vi "TrigerDelayer_测试Main.vi"() -> ()   [LabVIEW 2016]
uses:
  TrigerDelayer_ctl_TriggerSource.ctl
  Trigger Delayer.lvlib
panel:
  in  "Cluster":T2
  out "error out":errorcluster
  out "VISA resource name out":refnum<visa-resource-name>
  in  "VISA资源名称":refnum<visa-resource-name>
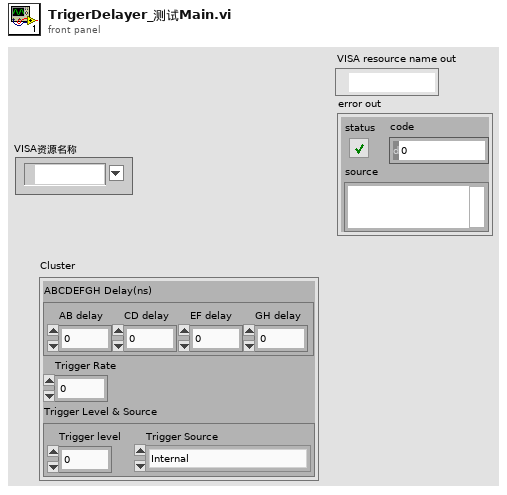
[diagram p1: front panel]
types:
  T1 = typedef "Trigger Delayer.lvlib/TrigerDelayer_ctl_TriggerSource.ctl" = enum16{"Internal", "External Rising Edges", "External Falling Edges", "Single Shot External Rising Edges", "Single Shot External Falling Edges", "Single Shot", "Line"}
  T2 = cluster{"ABCDEFGH Delay(ns)":cluster{"AB delay":dbl, "CD delay":dbl, "EF delay":dbl, "GH delay":dbl}, "Trigger Rate":dbl, "Trigger Level & Source":cluster{"Trigger level":dbl, "Trigger Source":T1}}
  T3 = cluster{"Trigger level":dbl, "Trigger Source":T1}
  T4 = cluster{"AB delay":dbl, "CD delay":dbl, "EF delay":dbl, "GH delay":dbl}
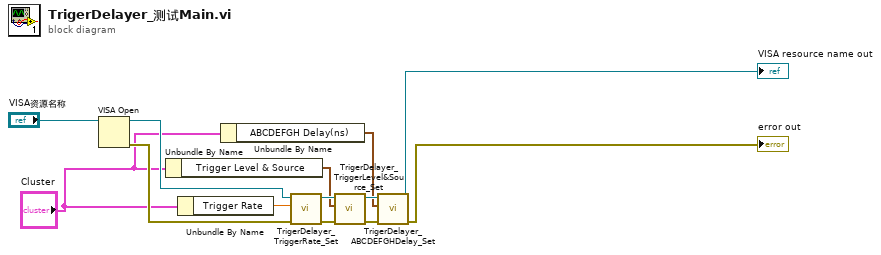
[diagram p0: block diagram]
diagram:
  n1 = VISA Open(VISA resource name="VISA资源名称") -> (VISA resource name=w12:refnum<visa-resource-name>, error out=w11:errorcluster)  [unwired: 4 in]
  n2 = Unbundle By Name("Cluster") -> ("Trigger Level & Source"=w3:T3)
  n3 = Unbundle By Name("Cluster") -> ("Trigger Rate"=w4:dbl)
  n4 = Unbundle By Name("Cluster") -> ("ABCDEFGH Delay(ns)"=w1:T4)
  n5 = call "TrigerDelayer_TriggerRate_Set.vi"("error in (no error)"=w11, "Trigger Rate"=w4, "VISA Refnum in"=w12) -> ("error out"=w9:errorcluster, "VISA Refnum out"=w10:refnum<visa-resource-name>)  [unwired: 7 in]
  n6 = call "TrigerDelayer_TriggerLevel&Source_Set.vi"("error in (no error)"=w9, "Trigger Level & Source"=w3, "VISA Refnum in"=w10) -> ("error out"=w6:errorcluster, "VISA Refnum out"=w8:refnum<visa-resource-name>)  [unwired: 7 in]
  n7 = call "TrigerDelayer_ABCDEFGHDelay_Set.vi"("error in (no error)"=w6, "ABCDEFGH Delay(ns)"=w1, "VISA Refnum in"=w8) -> ("error out"=→"error out":errorcluster, "VISA Refnum out"=→"VISA resource name out":refnum<visa-resource-name>)  [unwired: 7 in]
